vi "LED_Lights.vi"(0 "Dynamic Data 4":dynamicdata(waveform)) -> (20 "Amplitude":dynamicdata(waveform), 21 "Dynamic Data":dynamicdata(waveform), 22 "Amplitude 2":dynamicdata(waveform), 23 "Dynamic Data 2":dynamicdata(waveform), 24 "Amplitude 3":dynamicdata(waveform), 25 "Dynamic Data 3":dynamicdata(waveform))   [LabVIEW 2013]
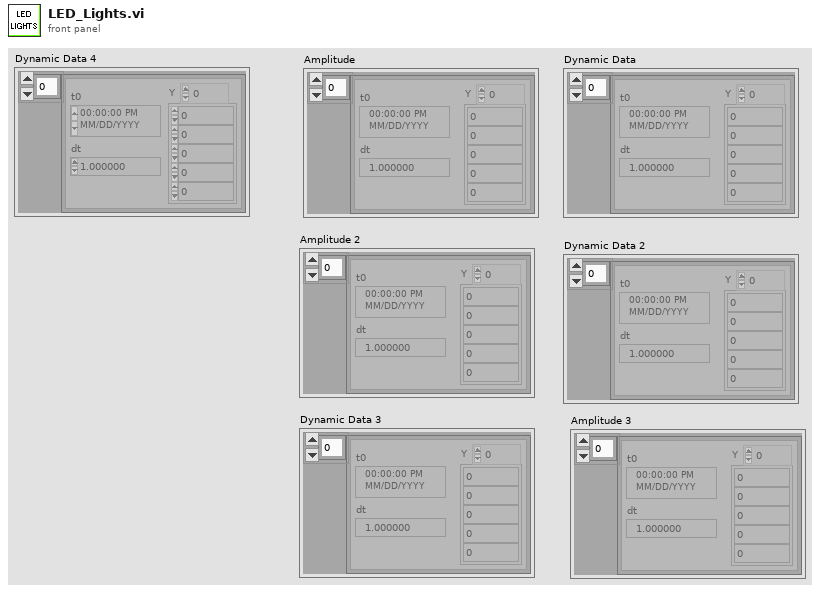
[diagram p1: front panel]
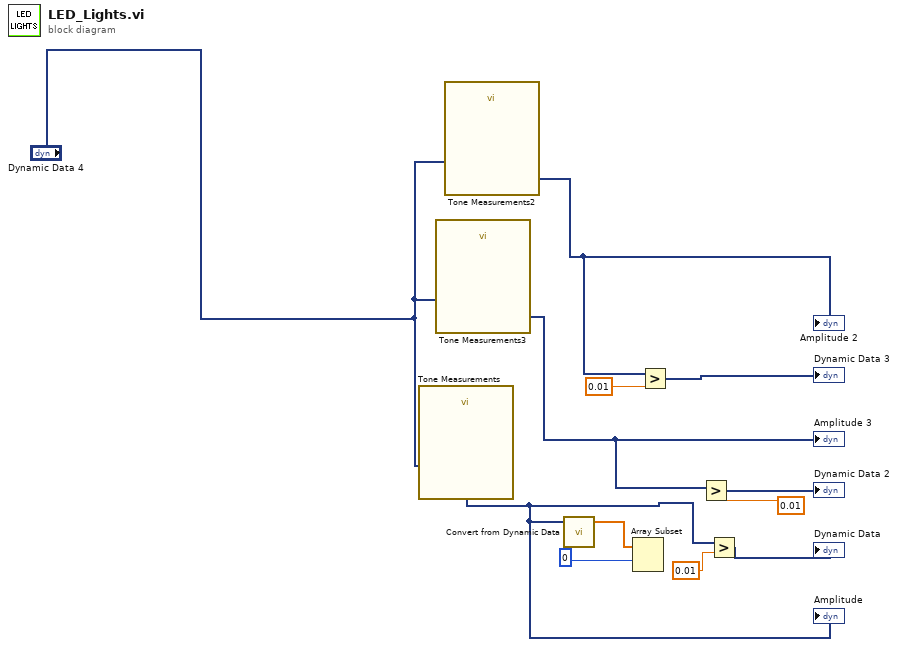
[diagram p0: block diagram]
diagram:
  n1 = call "Tone Measurements"("Signals"="Dynamic Data 4") -> ("Amplitude"=w12:dynamicdata)  [unwired: 9 in, 1 out]
  "Amplitude" <- w12
  n2 = call "Tone Measurements3"("Signals"="Dynamic Data 4") -> ("Amplitude"=w5:dynamicdata)  [unwired: 9 in, 1 out]
  "Amplitude 3" <- w5
  n3 = call "Tone Measurements2"("Signals"="Dynamic Data 4") -> ("Amplitude"=w6:dynamicdata)  [unwired: 9 in, 1 out]
  "Amplitude 2" <- w6
  n4 = call "Convert from Dynamic Data"("Dynamic Data Type"=w12) -> ("Array"=w9:dbl[])  [unwired: 3 in]
  n5 = Array Subset(array=w9, index=0) -> ()  [unwired: 1 in, 1 out]
  n6 = Greater?(x=w6, y=0.01) -> (0:→"Dynamic Data 3":dynamicdata)
  n7 = Greater?(x=w5, y=0.01) -> (0:→"Dynamic Data 2":dynamicdata)
  n8 = Greater?(x=w12, y=0.01) -> (0:→"Dynamic Data":dynamicdata)
